vi "Capacitance Configuration.vi"(8 "error in (no error)":errorcluster, 10 "Capacitance Range":T1, 11 "VISA resource name":refnum<visa-resource-name>) -> (0 "error out":errorcluster, 3 "VISA resource name out":refnum<visa-resource-name>)   [LabVIEW 2024, in "U1250 Series Digital Multimeter.lvlib"]
uses:
  <instrlib>/U1250 Series Multimeter Device Driver/U1250 Series Digital Multimeter.lvlib
  <instrlib>/U1250 Series Multimeter Device Driver/Controls/Capacitance Range.ctl
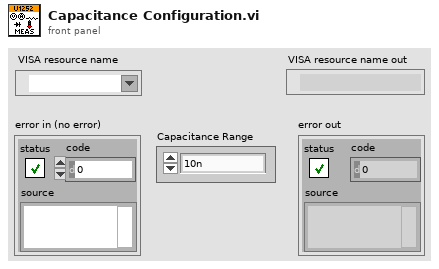
[diagram p1: front panel]
types:
  T1 = typedef "U1250 Series Digital Multimeter.lvlib/Capacitance Range.ctl" = enum16{"10n", "100n", "1000n", "10u", "100u", "1000u", "10m", "100m", "Auto"}
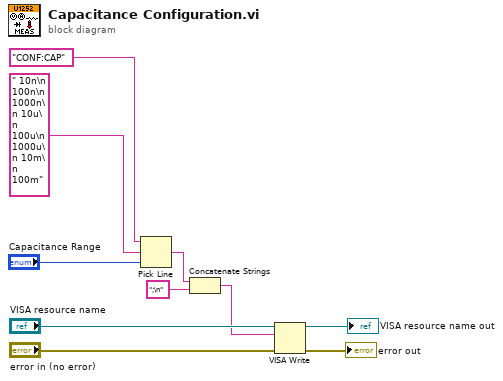
[diagram p0: block diagram]
diagram:
  n1 = Pick Line(string ("")="CONF:CAP", multi-line string=" 10n\n 100n\n 1000n\n 10u\n 100u\n 1000u\n 10m\n 100m", line index="Capacitance Range") -> (output string=w4:string)
  n2 = Concatenate Strings(w4, ";\n" ("string")) -> (w2:string)
  n3 = VISA Write(VISA resource name="VISA resource name", write buffer=w2, error in (no error)="error in (no error)") -> (VISA resource name out=→"VISA resource name out":refnum<visa-resource-name>, error out=→"error out":errorcluster)  [unwired: 1 out]
